vi "SetSettings.vi"(8 "error in (no error)":errorcluster, 9 "Value":string, 10 "Name":string) -> (0 "error out":errorcluster)   [LabVIEW 2017, in "Configuration.lvlib"]
doc: "Writes a value to the settings file."
uses:
  Configuration.lvlib
  <vilib>/Utility/config.llb/Write Key (String).vi
  <vilib>/Utility/config.llb/NI_LVConfig.lvlib
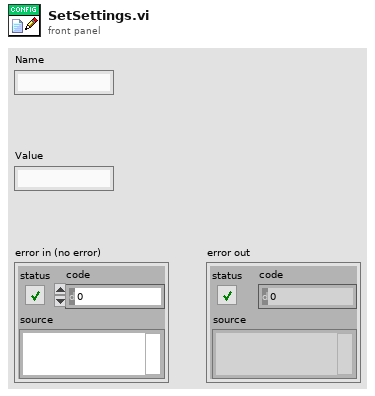
[diagram p1: front panel]
types:
  T1 = typedef "NI_LVConfig.lvlib/Config Data RefNum.ctl" = refnum<k1>
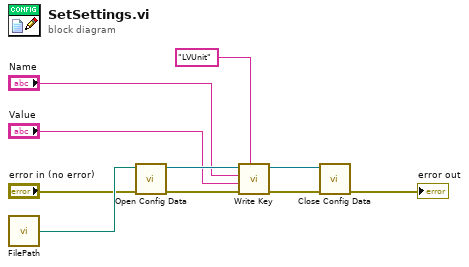
[diagram p0: block diagram]
diagram:
  n1 = call "FilePath.vi"() -> ("File Path"=w9:path)
  n2 = call <vilib>:"Open Config Data.vi"("error in (no error)"="error in (no error)", "configuration file path"=w9) -> ("error out"=w10:errorcluster, "refnum"=w6:T1)  [unwired: 7 in, 1 out]
  n3 = call-poly <vilib>:"Write Key.vi"("section"="LVUnit", "error in (no error)"=w10, "value"="Value", "key"="Name", "refnum"=w6) -> ("error out"=w8:errorcluster, "refnum out"=w5:T1)  [unwired: 4 in, 1 out]
  n4 = call <vilib>:"Close Config Data.vi"("error in (no error)"=w8, "refnum"=w5) -> ("error out"=→"error out":errorcluster)  [unwired: 8 in, 1 out]
